vi "Turn For Angle.vi"(0 "Speed":dbl, 2 "Description":string, 9 "Target Angle":dbl, 11 "Command Info In":T1, 12 "Synchronication":enum16{"Start", "Wait"}(ring)=enum."Wait") -> (4 "End Angle":dbl, 15 "Command Info Out":T1)   [LabVIEW 2017]
doc: "This VI notifies the subsystem to perform this command for the given duration, then go back to the default state. Synchronization determines whether this VI Starts the operation and returns immediately, or waits for the operation to complete. The first option is commonly used for TeleOp, and the second for Autonomous sequencing."
uses:
  <vilib>/Rock Robotics/WPI/Framework/Command Status Info.ctl
  <vilib>/Rock Robotics/WPI/Framework/Completion Status.ctl
  <vilib>/Rock Robotics/WPI/Framework/Completion Notifier.ctl
  Implementation/Drive Setpoints.ctl
  Implementation/Drive Operations.ctl
  Shared/RobotNeededPathData.ctl
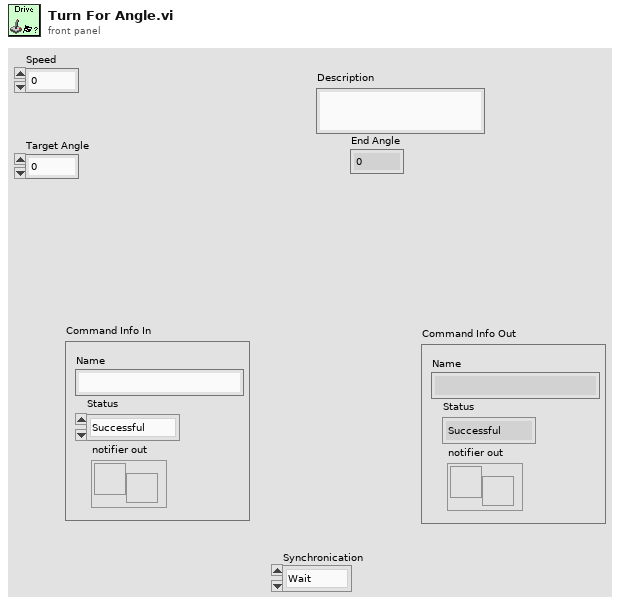
[diagram p1: front panel]
types:
  T1 = typedef "Command Status Info.ctl" = cluster{"Name":string, "Status":T2, "notifier out":T3}
  T2 = typedef "Completion Status.ctl" = enum16{"Successful", "Aborted", "Incomplete"}
  T3 = typedef "Completion Notifier.ctl" = refnum<notifier>
  T4 = typedef "Drive Setpoints.ctl" = cluster{"Operation":T5, "Left Speed":dbl, "Right Speed":dbl, "Duration":dbl, "Speed":dbl, "Start Angle":dbl, "Target Angle":dbl, "Distance (inch)":dbl, "Start Point (inch)":dbl, "RobotNeededPathData":T6, "Start Point 2":dbl}
  T5 = typedef "Drive Operations.ctl" = enum16{"Reserve", "Read Current", "Immediate", "Drive for Time", "Drive for Distance", "Turn to Angle", "Arc Turn", "Drive Path", "Drive To Cube"}
  T6 = typedef "RobotNeededPathData.ctl" = cluster{"Path":cluster{dbl, dbl}[], "MaxVel":dbl, "MaxAccel":dbl, "Backwards?":bool, "PointSpacing":dbl, "LookaheadDist":dbl, "Speed/Curve":dbl, "SlowDistanceAtEnd":dbl, "SlowSpeed":dbl}
  T7 = cluster{"Yaw":dbl, "Roll":dbl, "Pitch":dbl, "Heading":dbl, "Fused Heading":dbl}
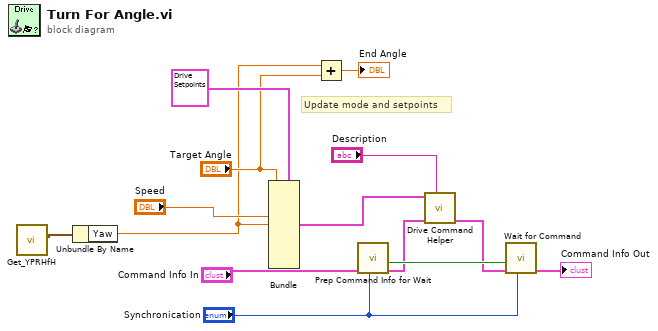
[diagram p0: block diagram]
diagram:
  # "Update mode and setpoints"
  n1 = call <vilib>:"Get_YPRHfH.vi"() -> ("YRPHfH"=w4:T7)  [unwired: 11 in]
  n2 = Unbundle By Name(w4) -> ("Yaw"=w2:dbl)
  n3 = Bundle(cluster=T4 {"Operation"=enum."Turn to Angle", "Left Speed"=0.0, "Right Speed"=0.0, "Duration"=0.0, "Speed"=0.0, "Start Angle"=0.0, "Target Angle"=0.0, "Distance (inch)"=0.0, "Start Point (inch)"=0.0, "RobotNeededPathData"={"Path"=[], "MaxVel"=0.0, "MaxAccel"=0.0, "Backwards?"=FALSE, "PointSpacing"=0.0, "LookaheadDist"=0.0, "Speed/Curve"=1.8, "SlowDistanceAtEnd"=12.0, "SlowSpeed"=15.0}, "Start Point 2"=0.0} ("SubSystem Data"), "Speed"="Speed", "Start Angle"=w2, "Target Angle"="Target Angle") -> (w7:T4)  [unwired: 8 in]
  n4 = Add(x=w2, y="Target Angle") -> (x+y=→"End Angle":dbl)
  n5 = call <vilib>:"Prep Command Info for Wait.vi"("Synchronication"="Synchronication", "Command Info"="Command Info In") -> ("Command Info"=w11:T1, "Allocated"=w12:bool)  [unwired: 8 in]
  n6 = call "Drive Command Helper.vi"("Description"="Description", "Command Info In"=w11, "SubSystem Data"=w7) -> ("Command Info Out"=w8:T1)  [unwired: 6 in, 2 out]
  n7 = call <vilib>:"Wait for Command.vi"("Synchronication"="Synchronication", "Command Info in"=w8, "Allocated"=w12) -> ("Command Info out"=→"Command Info Out":T1)  [unwired: 8 in]
